vi "test-SlippyInterval.vi"() -> ()   [LabVIEW 2021]
panel:
  in  "String":string
  out "Slip Count":i32
  in  "Pause":bool
  in  "Reset":bool
  in  "Interval (ms)":i32=1000
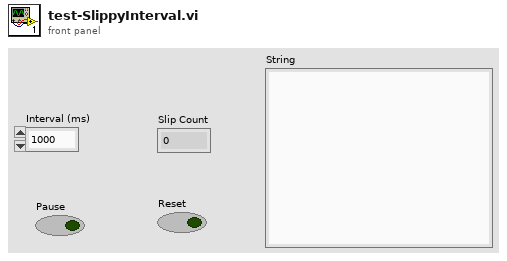
[diagram p1: front panel]
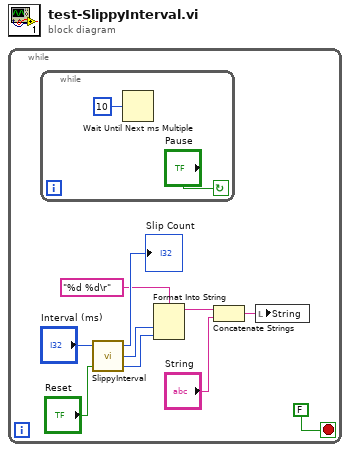
[diagram p0: block diagram]
diagram:
  n1 = while {
    stop <- FALSE stop-if-true
    n2 = while {
      stop <- "Pause" continue-if-true
      n3 = Wait Until Next ms Multiple(millisecond multiple=u32 10) -> ()  [unwired: 1 out]
    }
    n4 = call "SlippyInterval.vi"("Reset"="Reset", "Interval"="Interval (ms)") -> ("Next Interval (ms)"=w1:i32, "Elapsed Time (ms)"=w2:u32, "Slip Count"=→"Slip Count":i32)  [unwired: 1 in]
    n5 = Format Into String(format string="%d %d\r", w2, w1) -> (resulting string=w6:string)  [unwired: 2 in, 1 out]
    n6 = Concatenate Strings(w6, "String") -> (w7:string)
    n7 = local write "String"(w7) -> ()
  }
